vi "FFRS_SD.vi"   [LabVIEW 2015]
uses:
  DLL/ESLSCDLL.dll
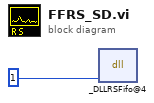
[diagram p0: block diagram]
diagram:
  n1 = dll-call lib="G:/SD/TRANCON-2015/DLL/ESLSCDLL.dll" fn="_DLLRSFifo@4" ("lwlscdll.dll:DLLRSFifo")("drv"=u32 1) -> ()  [unwired: 5 in, 2 out]
